vi "Remote Code to run.vi"(0 "Extra command String":string, 1 "Open Front Panel":bool, 2 "Raw data option":enum16{"Save raw data", "Raw data not saved"}(ring), 3 "Current Row Comments":string, 4 "Camera Resolution":T4=1 items=["Low", "Med.", "High", "Max."], 5 "setup":T3, 7 "Remote control":bool, 9 "File":T2, 11 "Results Filename":path, 12 "Raw data file":path, 13 "Averaging time (min)":dbl, 14 "Setup filename":string) -> (15 "Status":T1)   [LabVIEW 2022 SP3]
uses:
  Camera Server/Camera enum/Camera resolution.ctl
  Controls/Setup.ctl
  Controls/Save_Data.ctl
  Multi_Run_Status.ctl
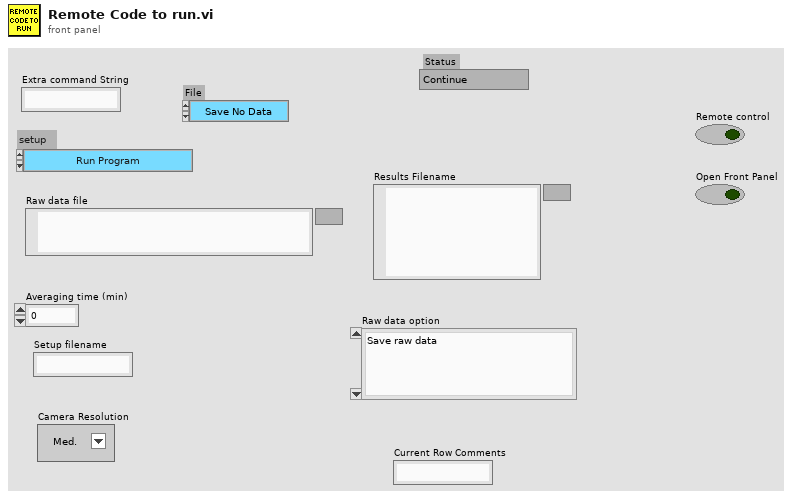
[diagram p1: front panel]
types:
  T1 = typedef "Multi_Run_Status.ctl" = enum16{"Continue", "Continue with Error", "Jump to Next Point", "Jump to Next Row", "Jump To Fall Back", "Terminate Run"}
  T2 = typedef "Save_Data.ctl" = enum16{"Save No Data", "Save Data"}
  T3 = typedef "Setup.ctl" = enum16{"Run Program", "Show Setup", "Save Current Setup", "Setup Front Panel"}
  T4 = typedef "Camera resolution.ctl" = u8
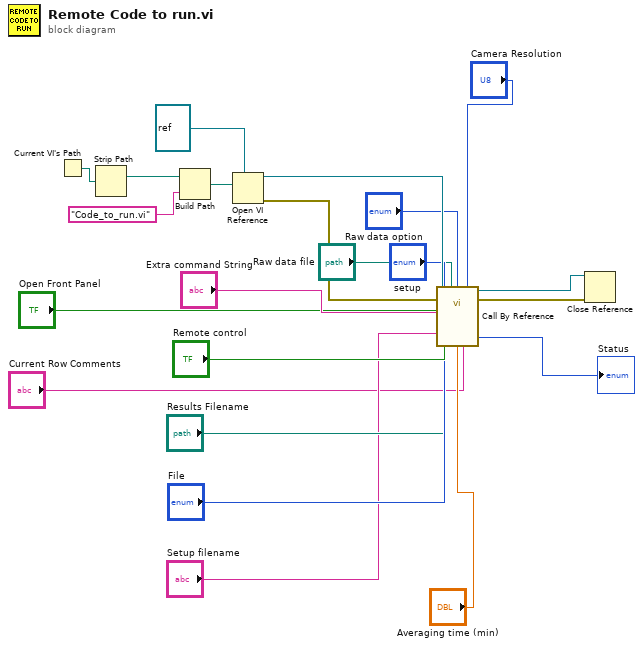
[diagram p0: block diagram]
diagram:
  n1 = Current VI's Path() -> (path=w4:path)
  n2 = Strip Path(path=w4) -> (stripped path=w2:path)  [unwired: 1 out]
  n3 = Build Path(base path=w2, name or relative path="Code_to_run.vi") -> (appended path=w1:path)
  n4 = Open VI Reference(type specifier VI Refnum (for type only)=refnum<vi> refnum ("Scout Server"), vi path=w1) -> (vi reference=w19:refnum<vi>, error out=w18:errorcluster)  [unwired: 2 in, 2 out]
  n5 = call-by-ref "?"(reference=w19, error in=w18, "Extra command String"="Extra command String", "Open Front Panel"="Open Front Panel", "Raw data option"="Raw data option", "Current Row Comments"="Current Row Comments", "Camera Resolution"="Camera Resolution", "setup"="setup", "Remote control"="Remote control", "File"="File", "Results Filename"="Results Filename", "Raw data file"="Raw data file", "Averaging time (min)"="Averaging time (min)", "Setup filename"="Setup filename") -> (reference out=w20:refnum<vi>, error out=w21:errorcluster, "Status"=→"Status":T1)  [unwired: 3 in]
  n6 = Close Reference(reference=w20, error in (no error)=w21) -> ()  [unwired: 1 out]
